vi "FPGA_DAC_move_2.vi"   [LabVIEW 2013]
uses:
  <vilib>/Platform/TimedLoop/XDataNode/timing_clust.ctl
  <vilib>/Platform/TimedLoop/XDataNode/nitl_modes.ctl
  <vilib>/Platform/TimedLoop/XDataNode/wakeup.ctl
  <vilib>/rvi/Emulation/niFpgaSctlEmulationGetInTimedLoop.vi
  <vilib>/rvi/Emulation/niFpgaEmulationReportErrorSimple.vi
  <vilib>/rvi/Emulation/niFpgaGetClockAttributes.vi
  <vilib>/rvi/FIFO/Fifo_Resource/nirvififoEmulationReadFpgaImpl.vi
  <vilib>/rvi/DataTransferAndStorage/Container/Common/niFpgaContainerGetUniqueNameForEmu.vi
  <vilib>/rvi/Emulation/niFpgaCriticalErrorInLSC.vi
  <vilib>/rvi/eio/common/nirviEmuTemplateMethod_errors.vi
  <vilib>/Platform/TimedLoop/XDataNode/XDataNode.xnode
  <vilib>/rvi/DataTransferAndStorage/Container/XNode/niFpgaContainer.xnode
  <vilib>/rvi/FIFO/Fifo_Resource/nirvififoEmulationRead.vi
  <vilib>/eio/EIONode/EIONode.xnode
  <vilib>/Platform/TimedLoop/XDataNode/XDNodeRunTimeDep.lvlib
types:
  T1 = typedef "XDNodeRunTimeDep.lvlib/timing_clust.ctl" = cluster{"Expected End [f-1]":u64, "Actual End [f-1]":u64, "Finished Late? [f-1]":bool, "Expected End [i-1]":u64, "Actual End [i-1]":u64, "Finished Late? [i-1]":bool, "Expected Start [i]":u64, "Actual Start [i]":u64, "Expected Start [f]":u64, "Actual Start [f]":u64, "Source Name":string, "Structure Name":string, "Period":i64, "Deadline":i64, "Offset":i64, "Start":i64, "Priority":i32, "Timeout":i32, "Mode":T2, "Wakeup Reason":T3, "Error":errorcluster, "Source Type":string, "Secondary Source Type":string, "Global End Time":u64, "Global Start Time":u64, "Frame Duration":u64, "Iteration Duration":u64, "Assigned CPU":i32, "I/O Scan Engine Mode":u32}
  T2 = typedef "XDNodeRunTimeDep.lvlib/nitl_modes.ctl" = enum32{"No Change", "Process missed periods, maintain original phase", "Discard missed periods, maintain original phase", "Process missed periods, ignore original phase", "Discard missed periods, ignore original phase"}
  T3 = typedef "XDNodeRunTimeDep.lvlib/wakeup.ctl" = enum32{"Normal", "Aborted", "Asynchronous wakeup", "Timing source error", "Timed loop error", "Timeout"}
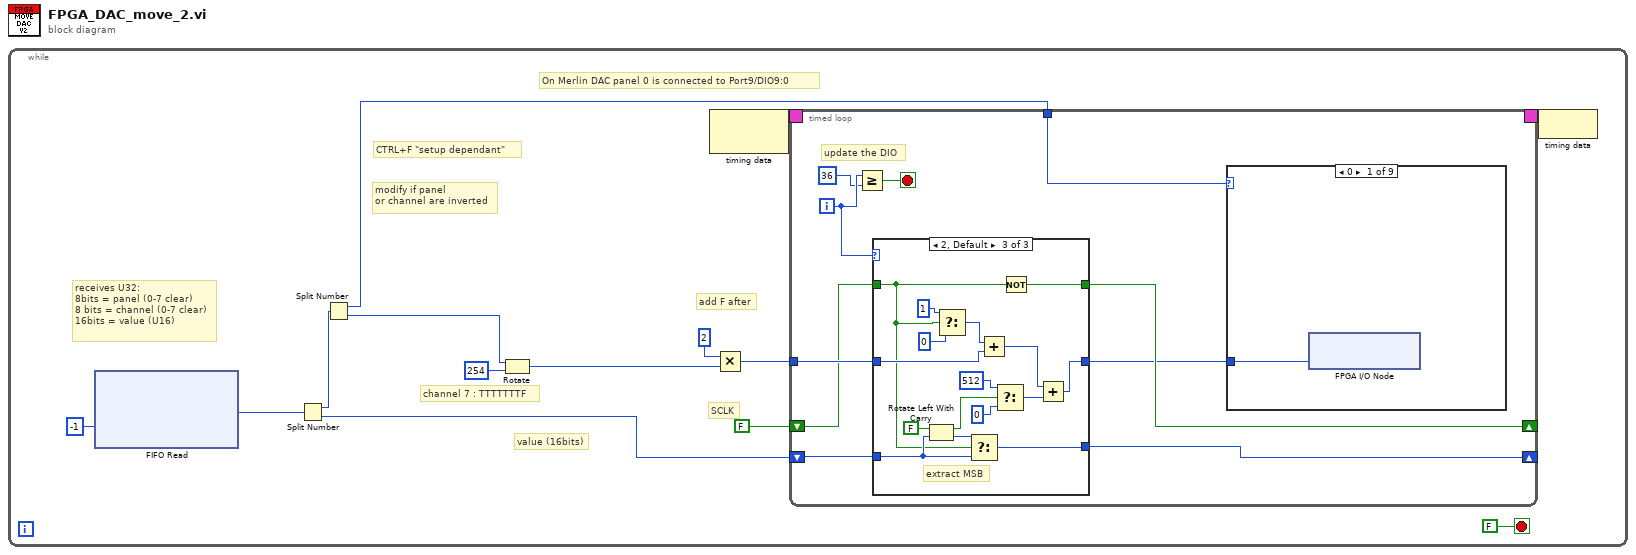
[diagram p0: block diagram]
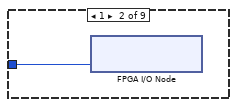
[diagram p2: hidden frame]
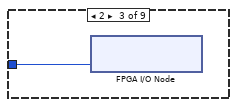
[diagram p3: hidden frame]
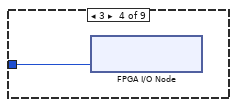
[diagram p4: hidden frame]
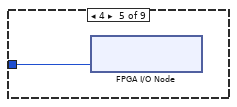
[diagram p5: hidden frame]
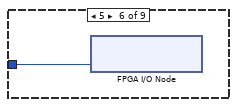
[diagram p6: hidden frame]
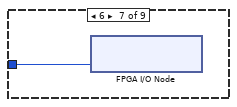
[diagram p7: hidden frame]
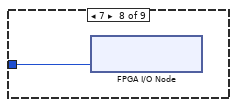
[diagram p8: hidden frame]
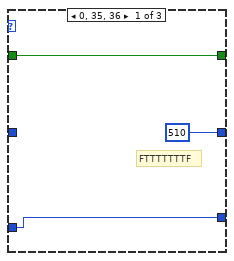
[diagram p10: hidden frame]
diagram:
  n1 = while {
    stop <- FALSE stop-if-true
    # "On Merlin DAC panel 0 is connected to Port9/DIO9:0"
    # "channel 7 : TTTTTTTF"
    # "add F after"
    # "SCLK"
    # "value (16bits)"
    # "modify if panel\nor channel are inverted"
    # "receives U32:\n8bits = panel (0-7 clear)\n8 bits = channel (0-7 clear)\n16bits = value (U16)"
    # "CTRL+F \"setup dependant\""
    n2 = xnode ("FIFO Read")("Timeout"=-1) -> ("Element"=w14:u32)  [unwired: 1 in, 2 out]
    n3 = Split Number(x=w14) -> (hi(x)=w13:u16, lo(x)=w12:u16)
    n4 = Split Number(x=w13) -> (hi(x)=w5:u8, lo(x)=w4:u8)
    n5 = Rotate(1:u8 254 ("x"), 2:w4) -> (0:w9:u8)
    n6 = node-c288() -> (w7:T1)  [unwired: 1 in]
    n7 = Multiply(x=u16 2 ("y"), y=w9) -> (x*y=w11:u16)
    n8 = timed-loop {
      tunnel: w11 -> [w23]
      shift-right: [w16] -> _
      shift-left: FALSE -> [w22]
      shift-right: [w21] -> _
      shift-left: w12 -> [w24]
      timing: w7 -> [_]
      timing-out: [_] -> w6
      tunnel: w5 -> [w20]
      i -> [w18]
      stop <- w19 stop-if-true
      # "update the DIO"
      n9 = Greater Or Equal?(x=w18, y=36) -> (x >= y?=w19:bool)
      n10 = case shown="2, Default" w18 {
        tunnel: [w35 w38 w54] -> w16
        tunnel: w24 -> [w34 w37 w53]
        tunnel: w23 -> [_ w36 w48]
        tunnel: w22 -> [w35 w38 w46]
        tunnel: [w34 w37 w45] -> w21
        tunnel: [u16 510 w36 w40] -> w15
        frame 0, 35, 36 {
          # "FTTTTTTTF"
        }
        frame 1, 34 {
        }
        frame 2, Default {
          # "extract MSB"
          n11 = Rotate Left With Carry(2:w53, 3:FALSE ("carry")) -> (0:w52:u16, 1:w39:bool)
          n12 = Select(t=u16 1, s=w46, f=u16 0 ("t")) -> (s? t:f=w49:u16)
          n13 = Select(t=w52, s=w46, f=w53) -> (s? t:f=w45:u16)
          n14 = Add(x=w49, y=w48) -> (x+y=w44:u16)
          n15 = Select(t=u16 512, s=w39, f=u16 0 ("t")) -> (s? t:f=w43:u16)
          n16 = Not(x=w46) -> (.not. x?=w54:bool)
          n17 = Add(x=w44, y=w43) -> (x+y=w40:u16)
        }
      }
      n18 = case shown="0" w20 {
        tunnel: w15 -> [w25 w26 w27 w28 w29 w30 w31 w32 _]
        frame 0 {
          n19 = xnode "FPGA I/O Node"("Port9/DIO9:0"=w25) -> ()  [unwired: 1 in, 1 out]
        }
        frame 1 {
          n20 = xnode "FPGA I/O Node"("Port8/DIO9:0"=w26) -> ()  [unwired: 1 in, 1 out]
        }
        frame 2 {
          n21 = xnode "FPGA I/O Node"("Port7/DIO9:0"=w27) -> ()  [unwired: 1 in, 1 out]
        }
        frame 3 {
          n22 = xnode "FPGA I/O Node"("Port6/DIO9:0"=w28) -> ()  [unwired: 1 in, 1 out]
        }
        frame 4 {
          n23 = xnode "FPGA I/O Node"("Port5/DIO9:0"=w29) -> ()  [unwired: 1 in, 1 out]
        }
        frame 5 {
          n24 = xnode "FPGA I/O Node"("Port4/DIO9:0"=w30) -> ()  [unwired: 1 in, 1 out]
        }
        frame 6 {
          n25 = xnode "FPGA I/O Node"("Port3/DIO9:0"=w31) -> ()  [unwired: 1 in, 1 out]
        }
        frame 7 {
          n26 = xnode "FPGA I/O Node"("Port2/DIO9:0"=w32) -> ()  [unwired: 1 in, 1 out]
        }
        frame 8, Default {
          # "not connected"
        }
      }
    }
    n27 = node-c288(w6) -> ()
  }
